vi "Mux I48xN.vi"(0 "i48xn in":fxp<+/-,48,0>[](array[numeric]), 5 "index":i32) -> (4 "i48 out":fxp<+/-,48,0>)   [LabVIEW 2017, in "Lock-In Amplifier Example FPGA.lvlib"]
uses:
  Lock-In Amplifier Example FPGA.lvlib
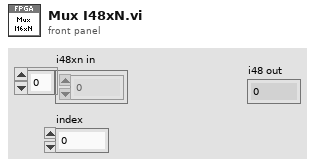
[diagram p1: front panel]
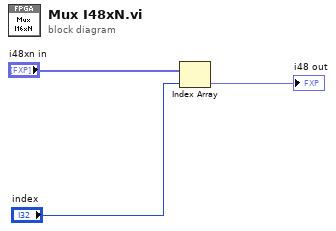
[diagram p0: block diagram]
diagram:
  n1 = Index Array(array="i48xn in", index="index") -> (element=→"i48 out":fxp<+/-,48,0>)
